vi "Errors.vi"   [LabVIEW 2017, in "DSF Core.lvlib" / "Dispatcher Interface.lvclass"]
uses:
  Dispatcher Interface.lvclass
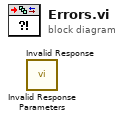
[diagram p0: block diagram]
diagram:
  n1 = call "Invalid Response Parameters.vi"() -> ()  [unwired: 10 in, 2 out]
  n2 = call "Invalid Response.vi"() -> ()  [unwired: 10 in, 2 out]
